vi "Arm.vi"() -> ()   [LabVIEW 2013]
uses:
  Globals/Homes.vi
  <vilib>/Rock Robotics/WPI/Joystick/WPI_JoystickGetSetRefNum.vi
  Robot Global Data.vi
  Globals/Auto.vi
  <vilib>/addons/control/pid/pid.llb/PID (DBL).vi
  Globals/Useful Values.vi
  Globals/Data for Dashboard.vi
  <vilib>/addons/control/pid/NI_PID_pid.lvlib
panel:
  out "UP?":bool=TRUE
  in  "PID gains DOWN":T1={"proportional gain (Kc)"=0.75, "integral time (Ti, min)"=0.0, "derivative time (Td, min)"=0.0} {"derivative time (Td, min)" format="%.3f"; "integral time (Ti, min)" format="%.3f"; "proportional gain (Kc)" format="%.3f"}
  out "Setpoint":dbl=0.8059999999999999
  out "Motor Output":dbl
  out "Arm Voltage":dbl=0.8012246490000001
  in  "PID gains UP":T1={"proportional gain (Kc)"=2.0, "integral time (Ti, min)"=0.0, "derivative time (Td, min)"=0.0} {"derivative time (Td, min)" format="%.3f"; "integral time (Ti, min)" format="%.3f"; "proportional gain (Kc)" format="%.3f"}
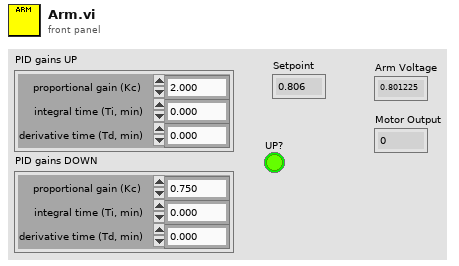
[diagram p1: front panel]
types:
  T1 = cluster{"proportional gain (Kc)":dbl, "integral time (Ti, min)":dbl, "derivative time (Td, min)":dbl}
  T2 = typedef "WPI_JoystickDevRef.ctl" = cluster{"Device":T3}
  T3 = typedef "WPI_JoystickDeviceEnum.ctl" = enum16{"USB 1", "USB 2", "USB 3", "USB 4", "Kinect 1", "Kinect 2"}
  T4 = typedef "WPI_AnalogChannelDevRef.ctl" = cluster{"DevStatus":errorcluster, "Analog Module":T5, "Analog Channel":T6}
  T5 = typedef "FPGA_TypedefAnalogModule.ctl" = enum16{"Analog Module 1", "Analog Module 2"}
  T6 = typedef "FPGA_AIChannel.ctl" = enum8{"AI 1", "AI 2", "AI 3", "AI 4", "AI 5", "AI 6", "AI 7", "AI 8", "Invalid"}
  T7 = typedef "WPI_MotorControlDeviceRef.ctl" = cluster{"DeviceStatus":errorcluster, "Type":enum16{"PWM", "CAN"}, "PWM":cluster{"Digital Module":T8, "PWM Channel":T9, "DeadBand":T10}, "CAN":cluster{"Device Number":u8, "Control Mode":T11, "Semaphore":T12, "Max Vout":dbl}, "Invert":bool, "TransformRef":T13, "InvTransformRef":T13}
  T8 = typedef "FPGA_TypedefDigitalModule.ctl" = enum16{"Digital Module 1", "Digital Module 2"}
  T9 = typedef "FPGA_DIOPWMChannel.ctl" = enum8{"PWM 1", "PWM 2", "PWM 3", "PWM 4", "PWM 5", "PWM 6", "PWM 7", "PWM 8", "PWM 9", "PWM 10", "Invalid"}
  T10 = typedef "WPI_PWMDeadband.ctl" = cluster{"Name":string, "maxPositivePwm":i32, "minPositivePwm":i32, "centerPwm":i32, "maxNegativePwm":i32, "minNegativePwm":i32, "angularRange":u16}
  T11 = typedef "WPI_CANJaguar_ControlMode.ctl" = enum8{"Percent VBus", "Current", "Speed", "Position", "Voltage"}
  T12 = typedef "Semaphore RefNum" = refnum<k1>
  T13 = typedef "WPI_PWMTransform_ConPane.ctl" = refnum<vi>
  T14 = typedef "WPI_DriverStationRobotMode2.ctl" = enum16{"Autonomous Disabled", "Autonomous Enabled", "Teleop Disabled", "Teleop Enabled", "Timeout", "Finish", "Test Disabled", "Test Enabled"}
  T15 = typedef "WPI_JoystickButtonState.ctl" = cluster{"Button 1":bool, "Button 2":bool, "Button 3":bool, "Button 4":bool, "Button 5":bool, "Button 6":bool, "Button 7":bool, "Button 8":bool, "Button 9":bool, "Button 10":bool, "Button 11":bool, "Button 12":bool}
  T16 = cluster{"axis 1 (x)":dbl, "axis 2 (y)":dbl, "axis 3 (throttle)":dbl, "axis 4":dbl, "axis 5":dbl, "axis 6":dbl}
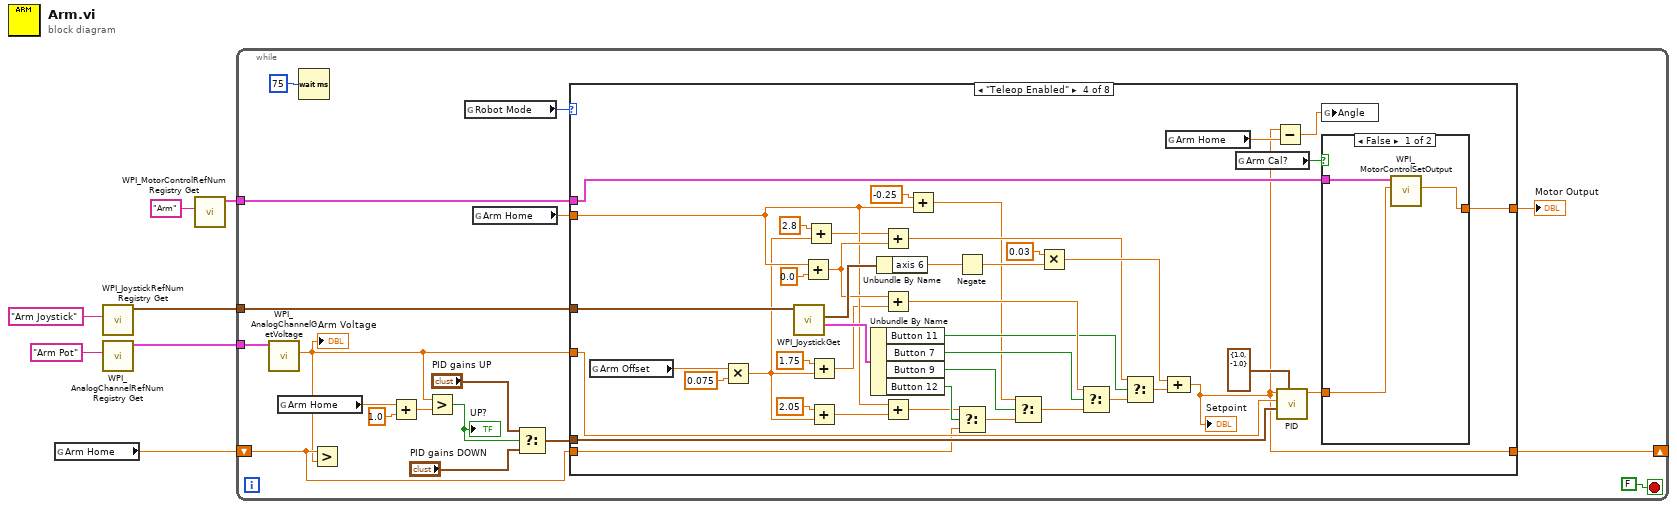
[diagram p0: block diagram]
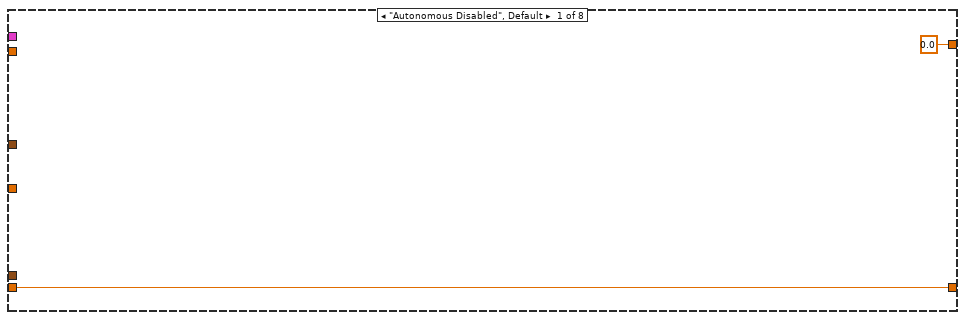
[diagram p2: hidden frame]
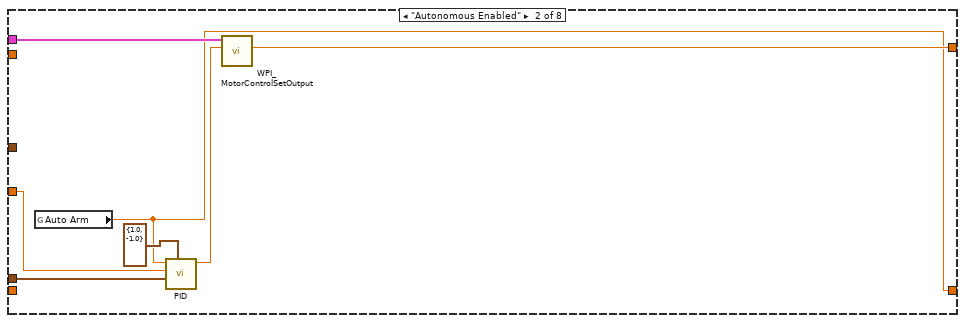
[diagram p3: hidden frame]
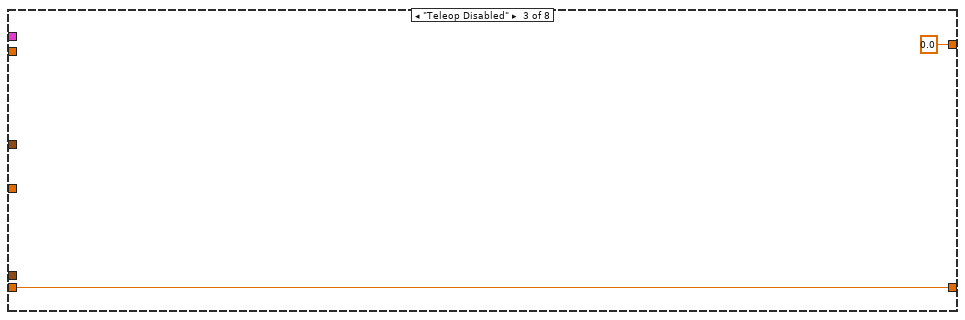
[diagram p4: hidden frame]
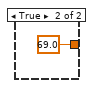
[diagram p5: hidden frame]
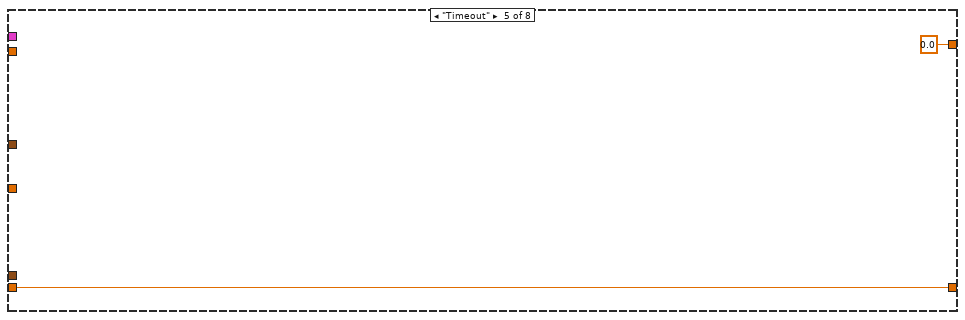
[diagram p6: hidden frame]
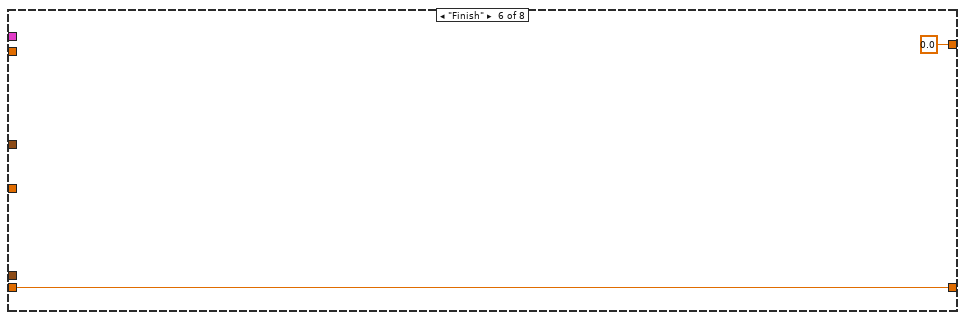
[diagram p7: hidden frame]
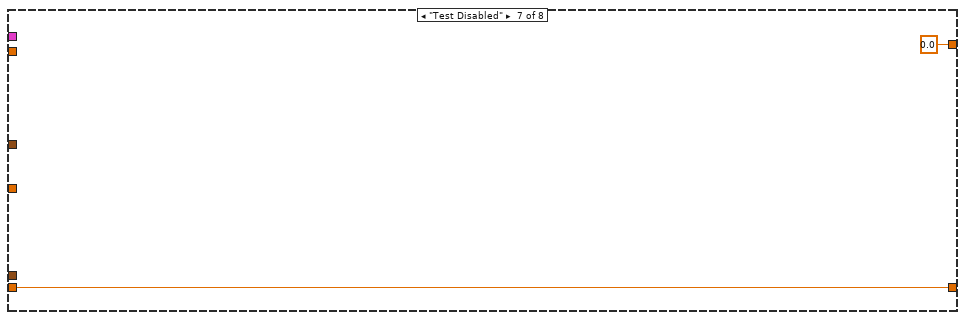
[diagram p8: hidden frame]
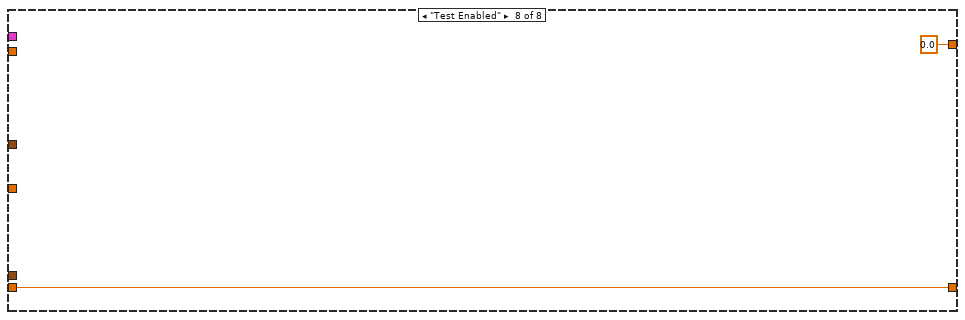
[diagram p9: hidden frame]
diagram:
  n1 = global read "Homes.vi" "Arm Home"() -> (w1:dbl)
  n2 = call <vilib>:"WPI_JoystickRefNum Registry Get.vi"("refnum name"="Arm Joystick") -> ("JoystickDevRef"=w2:T2)  [unwired: 9 in, 1 out]
  n3 = call <vilib>:"WPI_AnalogChannelRefNum Registry Get.vi"("refnum name"="Arm Pot") -> ("AIDeviceRef"=w7:T4)  [unwired: 9 in, 1 out]
  n4 = call <vilib>:"WPI_MotorControlRefNum Registry Get.vi"("refnum name"="Arm") -> ("MotorControlDevRef"=w4:T7)  [unwired: 9 in, 1 out]
  n5 = while {
    tunnel: w7 -> [w23]
    tunnel: w4 -> [w21]
    tunnel: w2 -> [w19]
    shift-right: [w18] -> _
    shift-left: w1 -> [w15]
    stop <- FALSE stop-if-true
    n6 = call <vilib>:"WPI_AnalogChannelGetVoltage.vi"("AIDeviceRef"=w23) -> ("Voltage"=w12:dbl)  [unwired: 8 in, 2 out]
    "Arm Voltage" <- w12
    n7 = global read "Homes.vi" "Arm Home"() -> (w11:dbl)
    n8 = Wait (ms)(milliseconds to wait=u32 75) -> ()  [unwired: 1 out]
    n9 = Greater?(x=w15, y=w12) -> ()  [unwired: 1 out]
    n10 = Add(x=w11, y=1.0) -> (x+y=w9:dbl)
    n11 = Greater?(x=w12, y=w9) -> (0:w13:bool)
    "UP?" <- w13
    n12 = global read "Robot Global Data.vi" "Robot Mode"() -> (w22:T14)
    n13 = global read "Homes.vi" "Arm Home"() -> (w8:dbl)
    n14 = Select(t="PID gains UP", s=w13, f="PID gains DOWN") -> (s? t:f=w14:T1)
    n15 = case shown="\"Teleop Enabled\"" w22 {
      tunnel: w21 -> [_ w33 _ w68 _ _ _ _]
      tunnel: w12 -> [_ w31 _ w71 _ _ _ _]
      tunnel: [0.0 ("Motor Output") w32 0.0 ("Motor Output") w66 0.0 ("Motor Output") 0.0 ("Motor Output") 0.0 ("Motor Output") 0.0 ("Motor Output")] -> w20
      tunnel: w19 -> [_ _ _ w78 _ _ _ _]
      tunnel: w8 -> [_ _ _ w48 _ _ _ _]
      tunnel: w15 -> [w26 _ w35 w52 w84 w86 w88 w90]
      tunnel: [w26 w30 w35 w45 w84 w86 w88 w90] -> w18
      tunnel: w14 -> [_ w28 _ w70 _ _ _ _]
      frame "Autonomous Disabled", Default {
      }
      frame "Autonomous Enabled" {
        n16 = global read "Auto.vi" "Auto Arm"() -> (w30:dbl)
        n17 = call-poly <vilib>:"PID.vi"("output range"=cluster{"output high":dbl, "output low":dbl} {"output high"=1.0, "output low"=-1.0}, "PID gains"=w28, "process variable"=w31, "setpoint"=w30) -> ("output"=w29:dbl)  [unwired: 6 in, 1 out]
        n18 = call <vilib>:"WPI_MotorControlSetOutput.vi"("Output"=w29, "MotorControlDevRef"=w33) -> ("Motor Output"=w32:dbl)  [unwired: 7 in, 2 out]
      }
      frame "Teleop Disabled" {
      }
      frame "Teleop Enabled" {
        n19 = global read "Useful Values.vi" "Arm Offset"() -> (w47:dbl)
        n20 = Multiply(x=w47, y=0.075) -> (x*y=w37:dbl)
        n21 = call <vilib>:"WPI_JoystickGet.vi"("JoystickDevRef"=w78) -> ("Buttons"=w77:T15, "Axes"=w65:T16)  [unwired: 4 in, 1 out]
        n22 = Add(x=w48, y=0.0) -> (x+y=w50:dbl)
        n23 = Add(x=2.8, y=w37) -> (x+y=w38:dbl)
        n24 = Add(x=1.75, y=w37) -> (x+y=w39:dbl)
        n25 = Add(x=2.05, y=w37) -> (x+y=w42:dbl)
        n26 = Unbundle By Name(w77) -> ("Button 11"=w58:bool, "Button 7"=w73:bool, "Button 9"=w72:bool, "Button 12"=w53:bool)
        n27 = Unbundle By Name(w65) -> ("axis 6"=w64:dbl)
        n28 = Add(x=w38, y=w50) -> (x+y=w57:dbl)
        n29 = Add(x=w50, y=w39) -> (x+y=w75:dbl)
        n30 = Add(x=w48, y=w42) -> (x+y=w51:dbl)
        n31 = Add(x=-0.25, y=w48) -> (x+y=w44:dbl)
        n32 = Negate(x=w64) -> (-x=w63:dbl)
        n33 = Select(t=w51, s=w53, f=w52) -> (s? t:f=w54:dbl)
        n34 = Select(t=w44, s=w72, f=w54) -> (s? t:f=w76:dbl)
        n35 = Multiply(x=0.03, y=w63) -> (x*y=w61:dbl)
        n36 = Select(t=w75, s=w73, f=w76) -> (s? t:f=w60:dbl)
        n37 = Select(t=w57, s=w58, f=w60) -> (s? t:f=w59:dbl)
        n38 = global read "Homes.vi" "Arm Home"() -> (w55:dbl)
        n39 = Compound Arithmetic op=ADD(w61, w59) -> (w45:dbl)
        "Setpoint" <- w45
        n40 = global read "Useful Values.vi" "Arm Cal?"() -> (w69:bool)
        n41 = Subtract(x=w45, y=w55) -> (x-y=w56:dbl)
        n42 = call-poly <vilib>:"PID.vi"("output range"=cluster{"output high":dbl, "output low":dbl} {"output high"=1.0, "output low"=-1.0}, "PID gains"=w70, "process variable"=w71, "setpoint"=w45) -> ("output"=w67:dbl)  [unwired: 6 in, 1 out]
        n43 = global write "Data for Dashboard.vi" "Angle"(w56) -> ()
        n44 = case shown="False" w69 {
          tunnel: w68 -> [w82 _]
          tunnel: w67 -> [w81 _]
          tunnel: [w80 69.0 ("Motor Output")] -> w66
          frame False {
            n45 = call <vilib>:"WPI_MotorControlSetOutput.vi"("Output"=w81, "MotorControlDevRef"=w82) -> ("Motor Output"=w80:dbl)  [unwired: 7 in, 2 out]
          }
          frame True {
          }
        }
      }
      frame "Timeout" {
      }
      frame "Finish" {
      }
      frame "Test Disabled" {
      }
      frame "Test Enabled" {
      }
    }
    "Motor Output" <- w20
  }
